vi "initialize_frontpanel.vi"(8 "error in (no error)":errorcluster, 11 "ColorOverlay in":refnum<class "ColorOverlay.lvclass">) -> (0 "error out":errorcluster, 3 "ColorOverlay out":refnum<class "ColorOverlay.lvclass">)   [LabVIEW 2010, in "ColorOverlay.lvclass"]
uses:
  ColorOverlay.lvclass
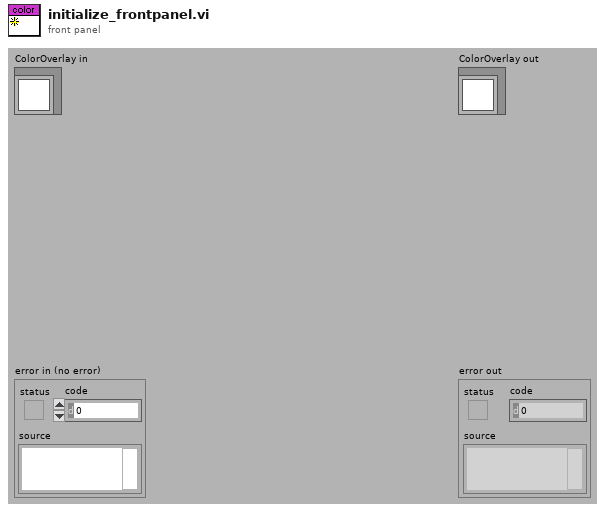
[diagram p1: front panel]
types:
  T1 = cluster{"Plot Name":string, "Plot Color":u32, "Plot Line Width":u8, "Plot Point Style":u8, "Plot Visible":bool}[]
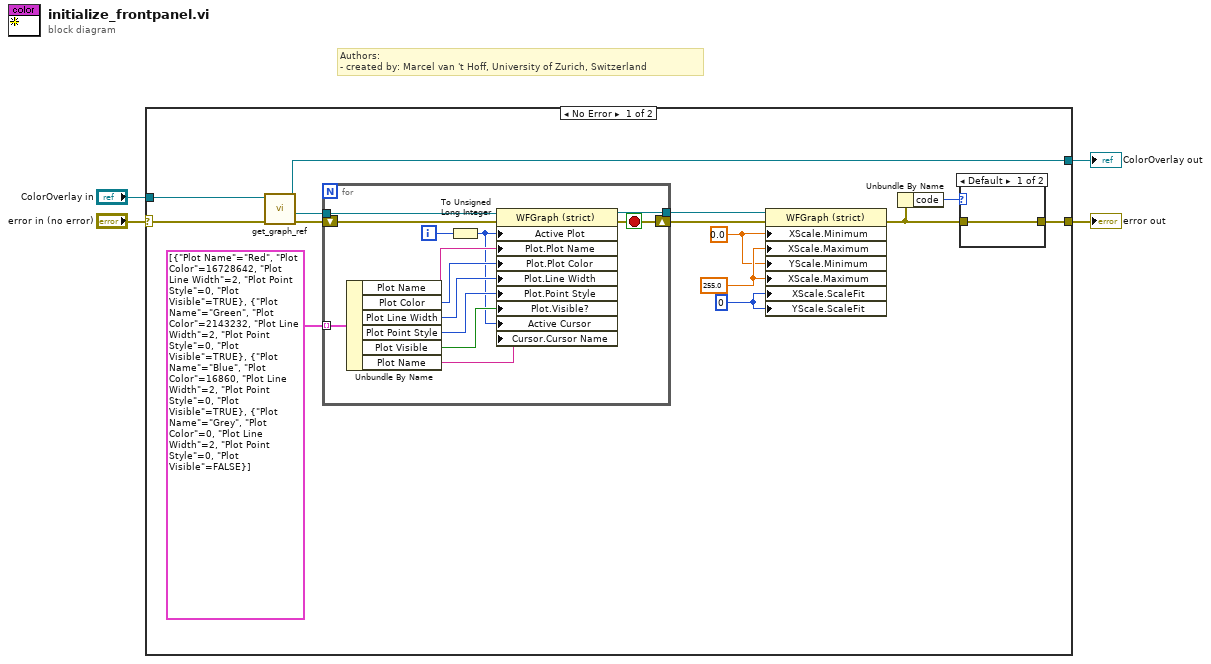
[diagram p0: block diagram]
diagram:
  # "Authors: \n- created by: Marcel van 't Hoff, University of Zurich, Switzerland"
  n1 = case shown="No Error" "error in (no error)" {
    selector: "error in (no error)" -> [w17 w34]
    tunnel: [w5 w34] -> w3
    tunnel: [w16 w33] -> w1
    tunnel: "ColorOverlay in" -> [w18 w33]
    frame No Error {
      w12 = 0.0 ("X Scale.Range:Maximum")
      w13 = 255.0 ("X Scale.Range:Maximum")
      w11 = u8 0 ("X Scale.Scale Fit")
      n2 = call-dynamic "get_graph_ref.vi"("error in (no error)"=w17, "ColorOverlay in"=w18) -> ("error out"=w9:errorcluster, "graph ref"=w8:refnum<vi>, "ColorOverlay out"=w16:refnum<class "ColorOverlay.lvclass">)  [unwired: 7 in]
      n3 = for {
        tunnel: w8 -> [w32]
        tunnel: T1 [{"Plot Name"="Red", "Plot Color"=16728642, "Plot Line Width"=2, "Plot Point Style"=0, "Plot Visible"=TRUE}, {"Plot Name"="Green", "Plot Color"=2143232, "Plot Line Width"=2, "Plot Point Style"=0, "Plot Visible"=TRUE}, {"Plot Name"="Blue", "Plot Color"=16860, "Plot Line Width"=2, "Plot Point Style"=0, "Plot Visible"=TRUE}, {"Plot Name"="Grey", "Plot Color"=0, "Plot Line Width"=2, "Plot Point Style"=0, "Plot Visible"=FALSE}] -> [w30] mode=indexing
        shift-right: [w21] -> w14
        shift-left: w9 -> [w22]
        tunnel: [w20] -> w15
        i -> [w31]
        stop <- w21 stop-if-true
        n4 = Unbundle By Name(w30) -> ("Plot Name"=w29:string, "Plot Color"=w28:u32, "Plot Line Width"=w27:u8, "Plot Point Style"=w26:u8, "Plot Visible"=w25:bool, "Plot Name"=w23:string)
        n5 = To Unsigned Long Integer(number=w31) -> (unsigned 32bit integer=w24:u32)
        n6 = property on="Property Node" class="WFGraph (strict)"(reference=w32, error in=w22, "Active Plot"=w24, "Plot.Plot Name"=w29, "Plot.Plot Color"=w28, "Plot.Line Width"=w27, "Plot.Point Style"=w26, "Plot.Visible?"=w25, "Active Cursor"=w24, "Cursor.Cursor Name"=w23) -> (reference out=w20:refnum<vi>, error out=w21:errorcluster)
      }
      n7 = property on="Property Node" class="WFGraph (strict)"(reference=w15, error in=w14, "XScale.Minimum"=w12, "XScale.Maximum"=w13, "YScale.Minimum"=w12, "XScale.Maximum"=w13, "XScale.ScaleFit"=w11, "YScale.ScaleFit"=w11) -> (error out=w6:errorcluster)  [unwired: 1 out]
      n8 = Unbundle By Name(w6) -> ("code"=w7:i32)
      n9 = case shown="Default" w7 {
        tunnel: w6 -> [w19 _]
        tunnel: [w19 _] -> w5
        frame Default {
        }
        frame 1077 {
        }
      }
    }
    frame Error {
    }
  }
  "error out" <- w3
  "ColorOverlay out" <- w1
